vi "Deferred Stop.vi"(10 "Log Instance":refnum<class "LoggerReference.lvclass">, 11 "Deferred Stop Time":u32) -> ()   [LabVIEW 2018, in "MVA Framework.lvlib" / "Composed Log.lvlib" / "LoggerReference.lvclass"]
uses:
  LoggerReference.lvclass
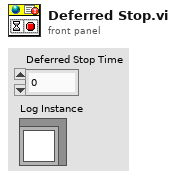
[diagram p1: front panel]
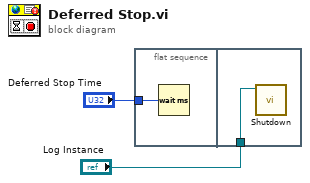
[diagram p0: block diagram]
diagram:
  n1 = flat-sequence {
    tunnel: "Deferred Stop Time" -> [w3]
    tunnel: "Log Instance" -> [w4]
    frame #0 {
      n2 = Wait (ms)(milliseconds to wait=w3) -> ()  [unwired: 1 out]
    }
    frame #1 {
      n3 = call "Shutdown.vi"("LoggerReference in"=w4) -> ()  [unwired: 10 in, 1 out]
    }
  }
